vi "Indexer.vi"() -> ()   [LabVIEW 2020]
doc: "Use this template to build a producer/consumer design pattern with events to produce queue items. Use this design pattern instead of the User Interface Event Handler pattern for user interfaces when you want to execute code asynchronously in response to an event without slowing the user interface responsiveness."
uses:
  Model/AbstractModel/AbstractModel.lvclass
  Model/MarkovModel/MarkovModel.lvclass
  C:/Projects/DMC/DMC-Complete/Model/AbstractModel/AbstractModel.lvclass
  Indexer Action.ctl
  File Metadata.ctl
  Node.ctl
  Source to Sink Array.ctl
  File Data.ctl
panel:
  out "data":T5
  in  "Tab Control":enum32{"Main", "Debug"}(tab)
  out "# of files":i32 format="%d files"
  out "Markov Progress":u64(slide) scale=-1.0..127701.0
  out "Saving model to file":bool
  in  "Run Training":bool
  in  "Training Folders":path[](array[path])
  in  "Load Example Paths":bool
  out "Pulling training files":bool
  out "Converting to node-child maps":bool
  out "Training model":bool
  out "Node Progress":u64(slide) scale=-1.0..1339.0
  in  "stop":bool
  in  "Load from file":bool
  in  "Save to file":bool
  in  "Stage 3 - Train Model":bool
  in  "Stage 1 - Pull Example Files":bool
  in  "Stage 2 - Convert to Node-Child Maps":bool
  in  "Parallel Instances":i32=8
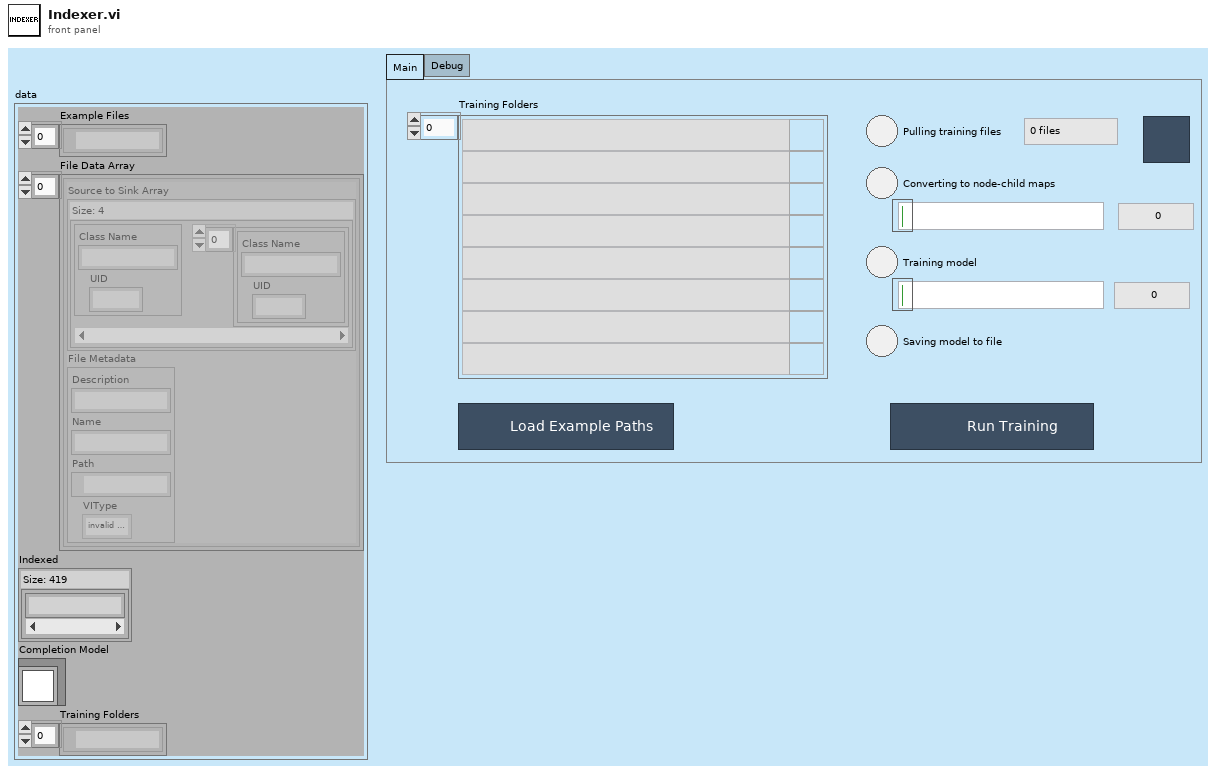
[diagram p1: front panel]
types:
  T1 = typedef "File Data.ctl" = cluster{"Source to Sink Array":T2, "File Metadata":T4}
  T2 = typedef "Source to Sink Array.ctl" = map{T3, T3[]}
  T3 = typedef "Node.ctl" = cluster{"Class Name":string, "UID":i32}
  T4 = typedef "File Metadata.ctl" = cluster{"Description":string, "Name":string, "Path":path, "VIType":enum32{"invalid VI type", "Standard VI", "Control VI", "Global VI", "Polymorphic VI", "Configuration VI", "SubSystem", "Facade VI", "Method VI", "Statechart Diagram VI"}}
  T5 = cluster{"Example Files":path[], "File Data Array":T1[], "Indexed":set{string}, "Completion Model":refnum<class "AbstractModel.lvclass">, "Training Folders":path[]}
  T6 = typedef "Indexer Action.ctl" = enum16{"Pull Training Files", "Convert to Node-Child Maps", "Train Model", "Save to file", "Load from file", "Load Example Paths"}
  T7 = enum8{"Enabled", "Disabled", "Disabled and Grayed Out"}
  T8 = cluster{"Example Files":path[], "File Data Array":T1[], "Indexed":set{string}, "MarkovModel out":refnum<class "MarkovModel.lvclass">, "Training Folders":path[]}
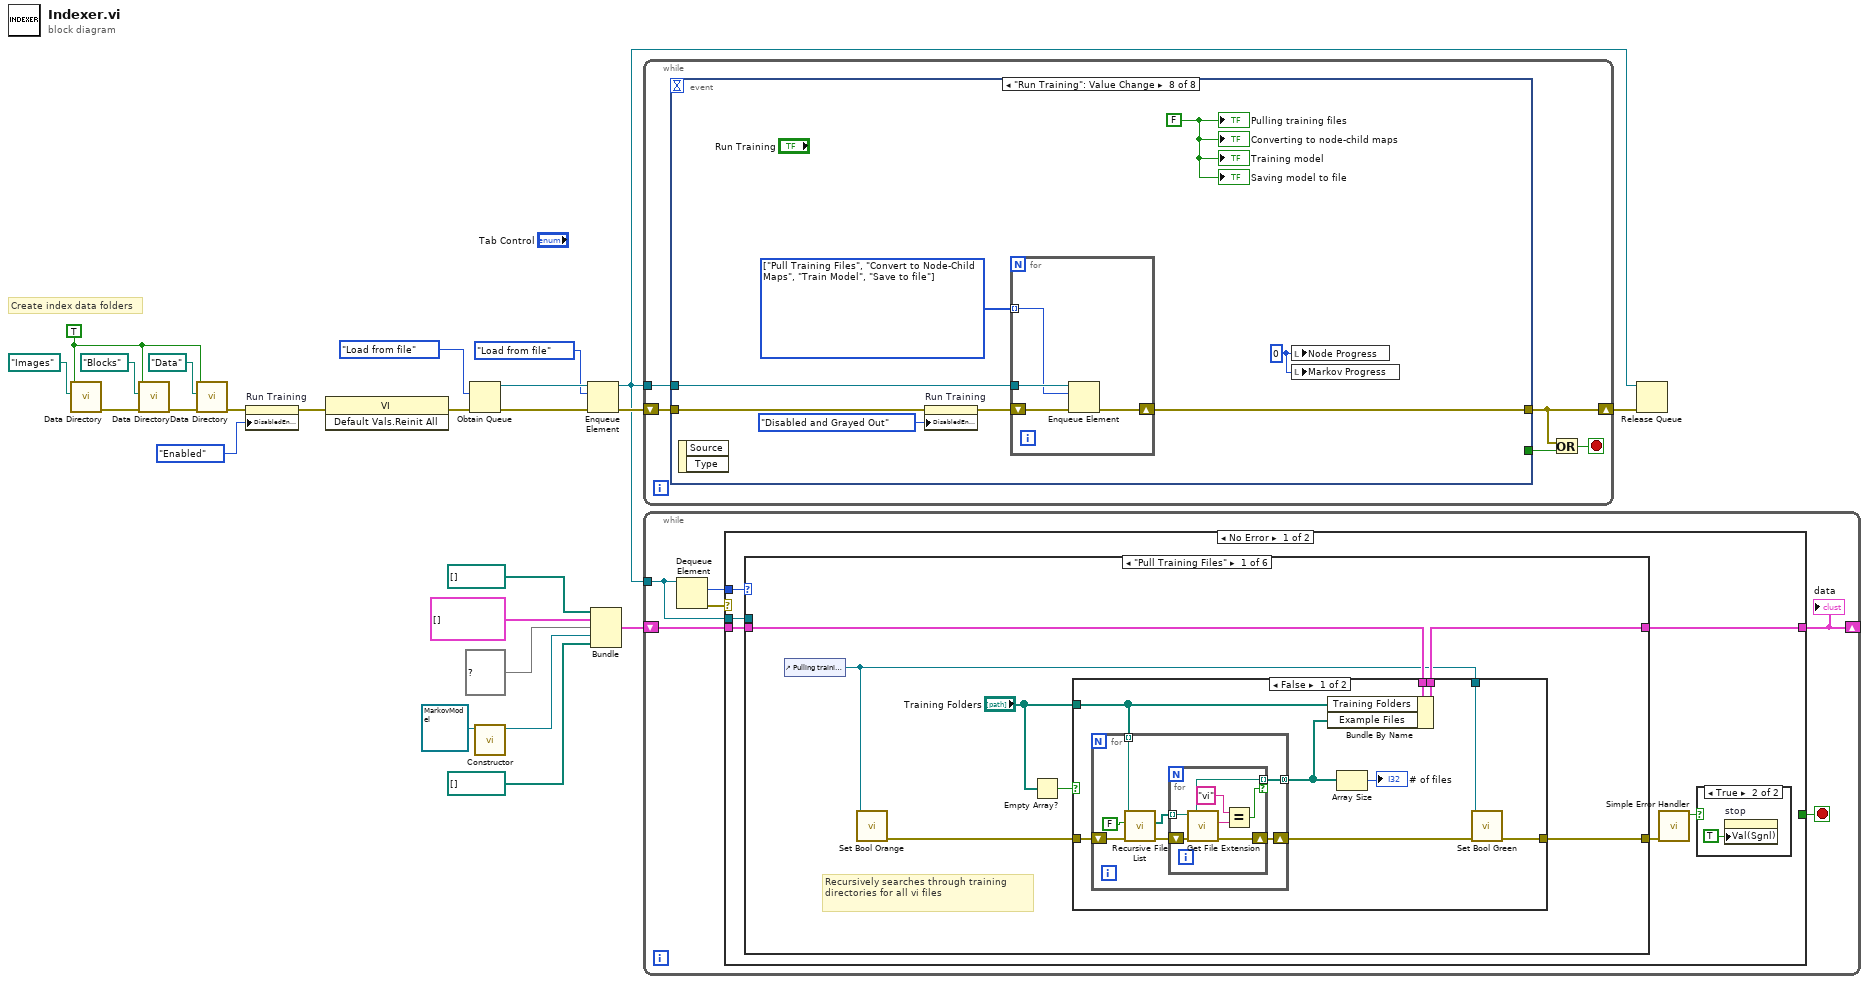
[diagram p0: block diagram]
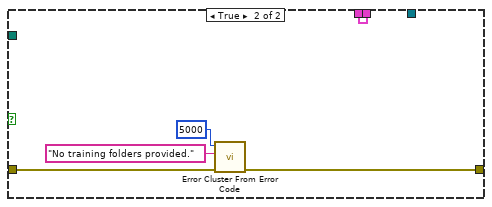
[diagram p2: hidden frame]
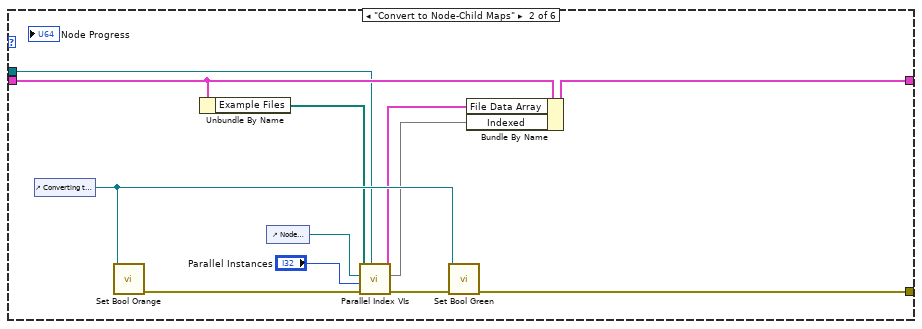
[diagram p3: hidden frame]
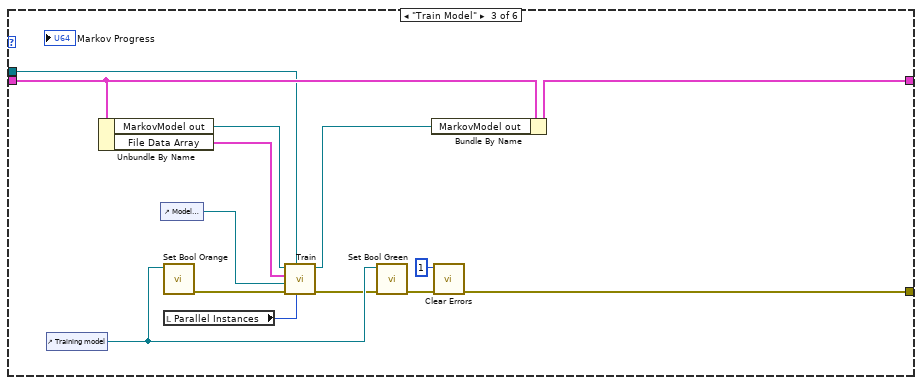
[diagram p4: hidden frame]
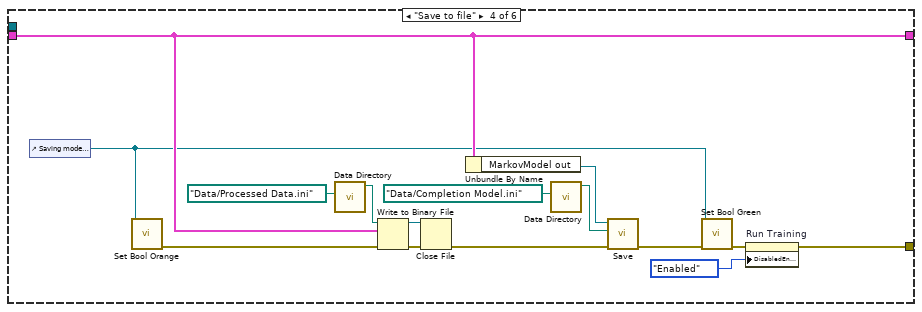
[diagram p5: hidden frame]
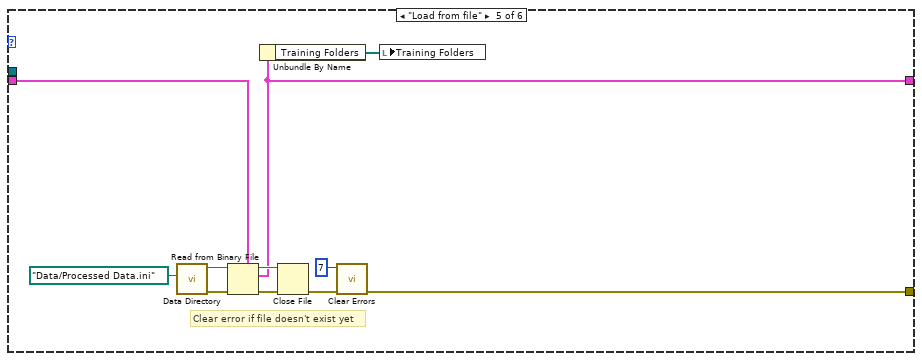
[diagram p6: hidden frame]
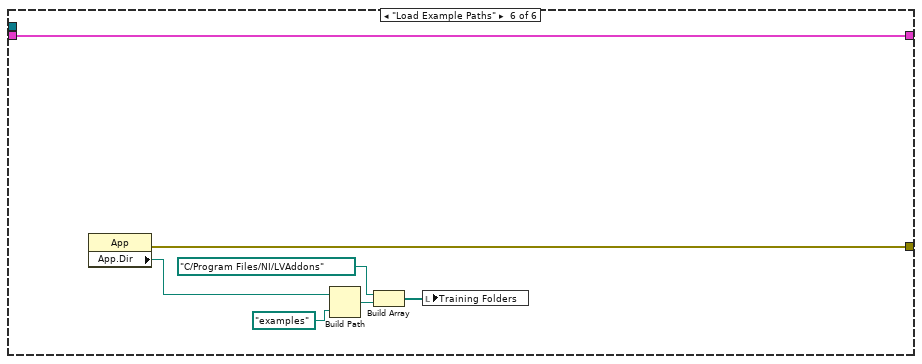
[diagram p7: hidden frame]
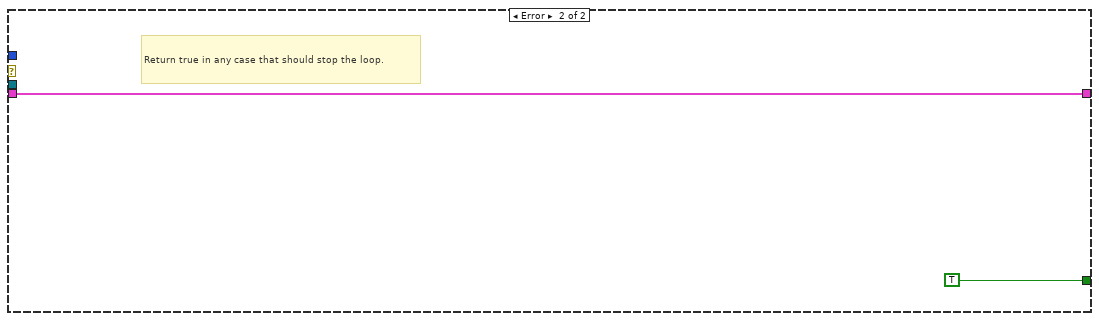
[diagram p9: hidden frame]
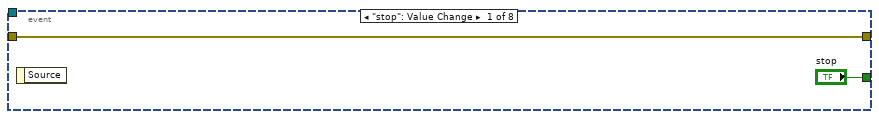
[diagram p10: hidden frame]
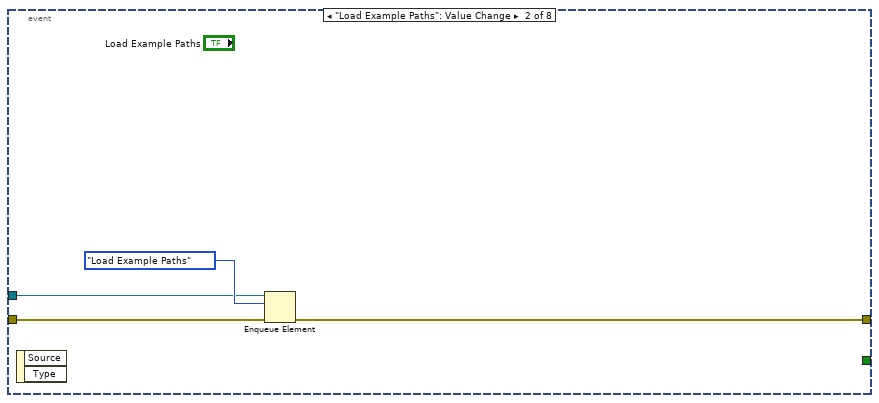
[diagram p11: hidden frame]
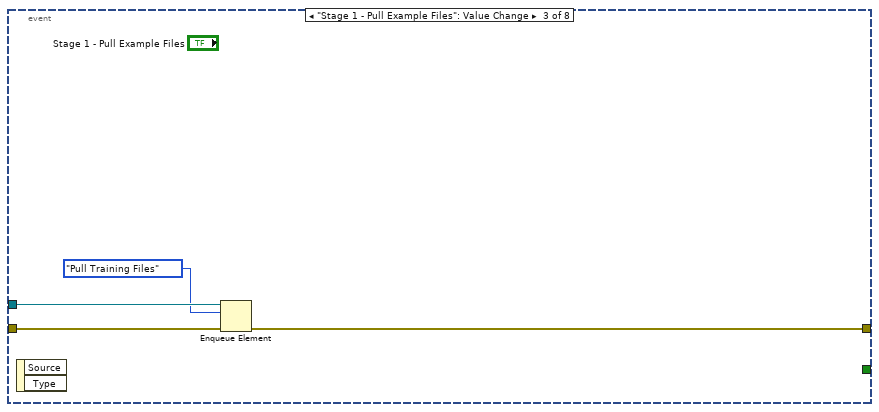
[diagram p12: hidden frame]
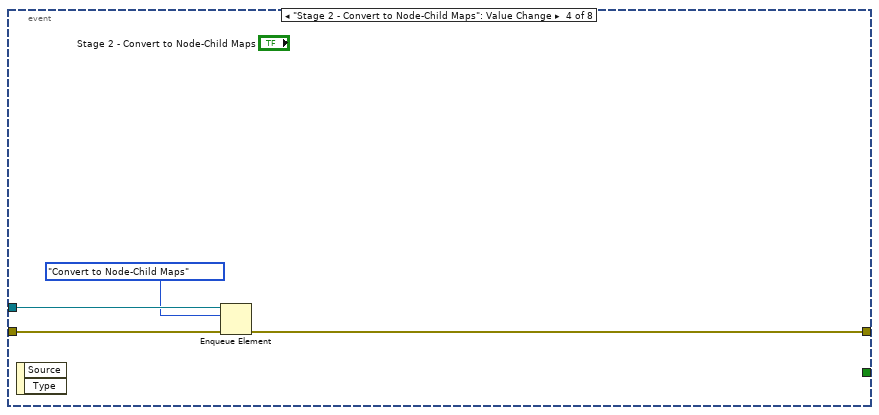
[diagram p13: hidden frame]
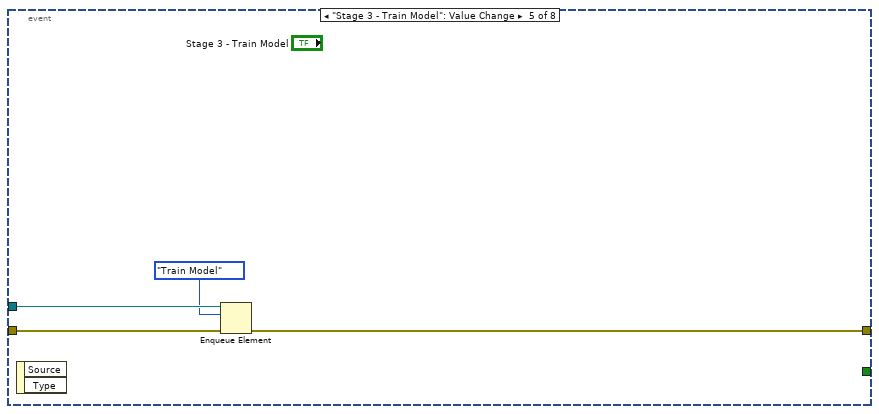
[diagram p14: hidden frame]
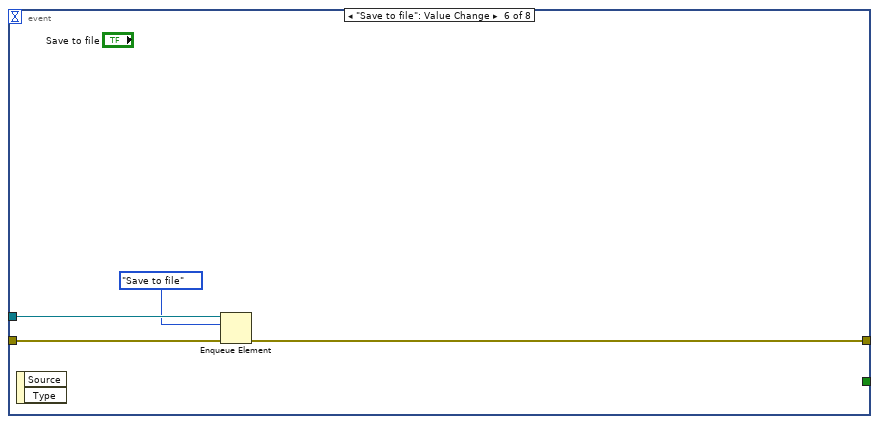
[diagram p15: hidden frame]
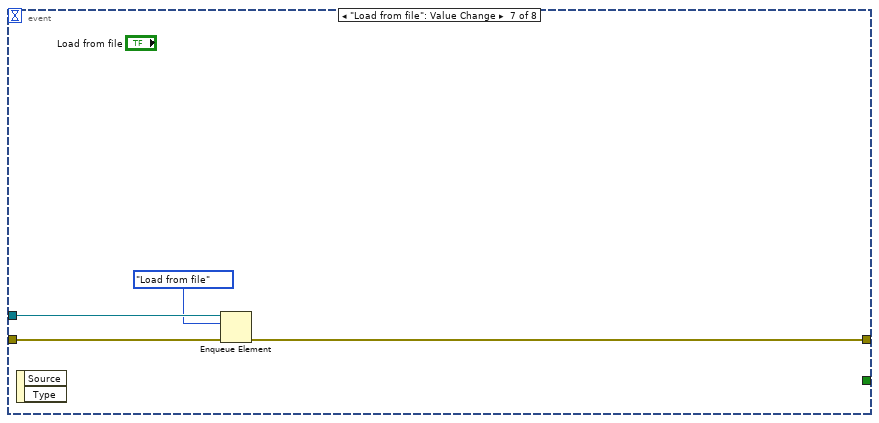
[diagram p16: hidden frame]
diagram:
  w5 = TRUE ("Create if doesn't exist? (F)")
  # "Create index data folders"
  n1 = call "Data Directory.vi"("Subdirectory"=path "Images" ("name or relative path"), "Create if doesn't exist? (F)"=w5) -> ("error out"=w6:errorcluster)  [unwired: 8 in, 1 out]
  n2 = call "Data Directory.vi"("error in (no error)"=w6, "Subdirectory"=path "Blocks" ("name or relative path"), "Create if doesn't exist? (F)"=w5) -> ("error out"=w7:errorcluster)  [unwired: 7 in, 1 out]
  n3 = call "Data Directory.vi"("error in (no error)"=w7, "Subdirectory"=path "Data" ("name or relative path"), "Create if doesn't exist? (F)"=w5) -> ("error out"=w4:errorcluster)  [unwired: 7 in, 1 out]
  n4 = property on="Run Training" class="Bool"(error in=w4, "DisabledEnum"=T7."Enabled") -> (error out=w12:errorcluster)  [unwired: 1 in, 1 out]
  n5 = invoke class="VI" method="Default Vals.Reinit All"(error in=w12) -> (error out=w14:errorcluster)  [unwired: 2 in, 2 out]
  n6 = Obtain Queue(element data type=Indexer_Action."Load from file" ("Indexer Action"), error in (no error)=w14) -> (queue out=w17:refnum<queue>, error out=w19:errorcluster)  [unwired: 3 in, 1 out]
  n7 = call-dynamic "Constructor.vi"("MarkovModel in"=refnum<class "MarkovModel.lvclass"> refnum ("MarkovModel.lvclass")) -> ("MarkovModel out"=w1:refnum<class "MarkovModel.lvclass">)  [unwired: 9 in, 1 out]
  n8 = Enqueue Element(queue=w17, element=Indexer_Action."Load from file", error in (no error)=w19) -> (queue out=w15:refnum<queue>, error out=w18:errorcluster)  [unwired: 1 in, 1 out]
  n9 = Bundle("Example Files"=path[] [], "File Data Array"=T1[] [], "Indexed"=set{string} {}, "MarkovModel out"=w1, "Training Folders"=path[] []) -> (w20:T8)  [unwired: 1 in]
  n10 = while {
    shift-right: [w25] -> w24
    shift-left: w18 -> [w28]
    tunnel: w15 -> [w29]
    stop <- w26 stop-if-true
    n11 = event shown="[7] \"Run Training\": Value Change" {
      selector: _ -> [_ _ _ _ _ _ _ _]
      dyn-events: _ -> [_ _ _ _ _ _ _ _]
      timeout: _ -> [_ _ _ _ _ _ _ _]
      tunnel: w29 -> [_ w32 w38 w42 w46 w50 w54 w63]
      tunnel: w28 -> [w30 w34 w39 w43 w47 w51 w55 w59]
      tunnel: [w30 w33 w37 w41 w45 w49 w53 w62] -> w25
      tunnel: ["stop" _ _ _ _ _ _ _] -> w27
      event "stop": Value Change {
        n12 = event-data() -> ()  [unwired: 1 in, 1 out]
      }
      event "Load Example Paths": Value Change {
        n13 = event-data() -> ()  [unwired: 1 in, 2 out]
        n14 = Enqueue Element(queue=w32, element=Indexer_Action."Load Example Paths" ("Indexer Action"), error in (no error)=w34) -> (error out=w33:errorcluster)  [unwired: 1 in, 2 out]
      }
      event "Stage 1 - Pull Example Files": Value Change {
        n15 = event-data() -> ()  [unwired: 1 in, 2 out]
        n16 = Enqueue Element(queue=w38, element=Indexer_Action."Pull Training Files" ("Indexer Action"), error in (no error)=w39) -> (error out=w37:errorcluster)  [unwired: 1 in, 2 out]
      }
      event "Stage 2 - Convert to Node-Child Maps": Value Change {
        n17 = event-data() -> ()  [unwired: 1 in, 2 out]
        n18 = Enqueue Element(queue=w42, element=Indexer_Action."Convert to Node-Child Maps" ("Indexer Action"), error in (no error)=w43) -> (error out=w41:errorcluster)  [unwired: 1 in, 2 out]
      }
      event "Stage 3 - Train Model": Value Change {
        n19 = event-data() -> ()  [unwired: 1 in, 2 out]
        n20 = Enqueue Element(queue=w46, element=Indexer_Action."Train Model" ("Indexer Action"), error in (no error)=w47) -> (error out=w45:errorcluster)  [unwired: 1 in, 2 out]
      }
      event "Save to file": Value Change {
        n21 = event-data() -> ()  [unwired: 1 in, 2 out]
        n22 = Enqueue Element(queue=w50, element=Indexer_Action."Save to file" ("Indexer Action"), error in (no error)=w51) -> (error out=w49:errorcluster)  [unwired: 1 in, 2 out]
      }
      event "Load from file": Value Change {
        n23 = event-data() -> ()  [unwired: 1 in, 2 out]
        n24 = Enqueue Element(queue=w54, element=Indexer_Action."Load from file" ("Indexer Action"), error in (no error)=w55) -> (error out=w53:errorcluster)  [unwired: 1 in, 2 out]
      }
      event "Run Training": Value Change {
        w56 = u64 0 ("Node Progress")
        w57 = FALSE ("Pulling training files")
        w61 = T6[] [enum."Pull Training Files", enum."Convert to Node-Child Maps", enum."Train Model", enum."Save to file"] items=["Pull Training Files", "Convert to Node-Child Maps", "Train Model", "Save to file", "Load from file", "Load Example Paths"] ("Array")
        n25 = event-data() -> ()  [unwired: 1 in, 2 out]
        n26 = property on="Run Training" class="Bool"(error in=w59, "DisabledEnum"=T7."Disabled and Grayed Out" ("Disabled")) -> (error out=w60:errorcluster)  [unwired: 1 in, 1 out]
        n27 = for {
          tunnel: w63 -> [w66]
          tunnel: w61 -> [w64] mode=indexing
          shift-right: [w65] -> w62
          shift-left: w60 -> [w67]
          n28 = Enqueue Element(queue=w66, element=w64, error in (no error)=w67) -> (error out=w65:errorcluster)  [unwired: 1 in, 2 out]
        }
        n29 = local write "Node Progress"(w56) -> ()
        n30 = local write "Markov Progress"(w56) -> ()
        "Converting to node-child maps" <- w57
        "Training model" <- w57
        "Pulling training files" <- w57
        "Saving model to file" <- w57
      }
    }
    n31 = Or(x=w25, y=w27) -> (x .or. y?=w26:bool)
  }
  n32 = while {
    tunnel: w15 -> [w69]
    shift-right: [w68] -> _
    shift-left: w20 -> [w70]
    stop <- w71 stop-if-true
    n33 = Dequeue Element(queue=w69) -> (element=w72:T6, error out=w73:errorcluster)  [unwired: 2 in, 2 out]
    n34 = case shown="No Error" w73 {
      tunnel: w72 -> [w79 _]
      tunnel: [_ TRUE] -> w71
      tunnel: w70 -> [w78 w174]
      tunnel: [w77 w174] -> w68
      tunnel: w69 -> [w76 _]
      frame No Error {
        n35 = case shown="\"Pull Training Files\"" w79 {
          tunnel: [w85 w125 w139 w152 w155 w167] -> w77
          tunnel: w78 -> [w86 w124 w137 w152 w163 w167]
          tunnel: w76 -> [_ w118 w131 _ _ _]
          tunnel: [w83 w122 w135 w147 w157 w168] -> w75
          frame "Pull Training Files" {
            # "Recursively searches through training directories for all vi files"
            n36 = control-ref of="Pulling training files"() -> (w82:refnum<vi>)
            n37 = call "Set Bool Orange.vi"("Indicator ref in"=w82) -> ("error out"=w84:errorcluster)  [unwired: 10 in]
            n38 = Empty Array?(array="Training Folders") -> (empty?=w80:bool)
            n39 = case shown="False" w80 {
              tunnel: w86 -> [w95 w113]
              tunnel: [w94 w113] -> w85
              tunnel: w84 -> [w93 w112]
              tunnel: [w91 w111] -> w83
              tunnel: w82 -> [w90 _]
              tunnel: "Training Folders" -> [w87 _]
              frame False {
                n40 = for {
                  tunnel: w87 -> [w102] mode=indexing
                  shift-right: [w97] -> w92
                  shift-left: w93 -> [w98]
                  tunnel: [w96] -> w89 mode=concatenating
                  n41 = call <vilib>:"Recursive File List.vi"("error in (no error)"=w98, "Treat LLBs as Folders?"=FALSE, "Folder Path"=w102) -> ("error out"=w99:errorcluster, "All Files in Dir"=w100:path[])  [unwired: 4 in, 3 out]
                  n42 = for {
                    tunnel: w100 -> [w105] mode=indexing
                    tunnel: [w105] -> w96 mode=indexing if=w104
                    shift-right: [w103] -> w97
                    shift-left: w99 -> [w108]
                    n43 = call <vilib>:"Get File Extension.vi"("error in (no error)"=w108, "file"=w105) -> ("error out"=w103:errorcluster, "lowercase file extension"=w106:string)  [unwired: 5 in, 3 out]
                    n44 = Equal?(x="vi", y=w106) -> (x = y?=w104:bool)
                  }
                }
                n45 = Bundle By Name(cluster=w95, "Training Folders"=w87, "Example Files"=w89) -> (w94:T8)
                n46 = Array Size(array=w89) -> (size(s)=→"# of files":i32)
                n47 = call "Set Bool Green.vi"("error in (no error)"=w92, "Indicator ref in"=w90) -> ("error out"=w91:errorcluster)  [unwired: 9 in]
              }
              frame True {
                n48 = call <vilib>:"Error Cluster From Error Code.vi"("error in (no error)"=w112, "error message (\"\")"="No training folders provided." ("error message (\"\")"), "error code (0)"=5000) -> ("error out"=w111:errorcluster)  [unwired: 6 in]
              }
            }
          }
          frame "Convert to Node-Child Maps" {
            n49 = control-ref of="Converting to node-child maps"() -> (w121:refnum<vi>)
            n50 = call "Set Bool Orange.vi"("Indicator ref in"=w121) -> ("error out"=w123:errorcluster)  [unwired: 10 in]
            n51 = Unbundle By Name(w124) -> ("Example Files"=w119:path[])
            n52 = control-ref of="Node Progress"() -> (w117:refnum<vi>)
            n53 = call "Parallel Index VIs.vi"("Queue in"=w118, "error in (no error)"=w123, "Parallel Instances (8)"="Parallel Instances", "Node Progress ref"=w117, "Example Files"=w119) -> ("error out"=w120:errorcluster, "Indexed"=w116:set{string}, "File Data Array"=w114:T1[])  [unwired: 4 in]
            n54 = call "Set Bool Green.vi"("error in (no error)"=w120, "Indicator ref in"=w121) -> ("error out"=w122:errorcluster)  [unwired: 9 in]
            n55 = Bundle By Name(cluster=w124, "File Data Array"=w114, "Indexed"=w116) -> (w125:T8)
          }
          frame "Train Model" {
            n56 = control-ref of="Training model"() -> (w138:refnum<vi>)
            n57 = Unbundle By Name(w137) -> ("MarkovModel out"=w130:refnum<class "MarkovModel.lvclass">, "File Data Array"=w129:T1[])
            n58 = control-ref of="Model Progress"() -> (w128:refnum<vi>)
            n59 = call "Set Bool Orange.vi"("Indicator ref in"=w138) -> ("error out"=w133:errorcluster)  [unwired: 10 in]
            n60 = local read "Parallel Instances"() -> (w127:i32)
            n61 = call-dynamic "Train.vi"("Parallel Instances (8)"=w127, "Queue in"=w131, "error in (no error)"=w133, "Progress ref in"=w128, "File Data Array"=w129, "MarkovModel in"=w130) -> ("error out"=w132:errorcluster, "MarkovModel out"=w126:refnum<class "MarkovModel.lvclass">)  [unwired: 4 in]
            n62 = call "Set Bool Green.vi"("error in (no error)"=w132, "Indicator ref in"=w138) -> ("error out"=w136:errorcluster)  [unwired: 9 in]
            n63 = Bundle By Name(cluster=w137, "MarkovModel out"=w126) -> (w139:T8)
            n64 = call <vilib>:"Clear Errors.vi"("error in (no error)"=w136, "specific error code to clear (0: all)"=1) -> ("error out"=w135:errorcluster)  [unwired: 4 in, 1 out]
          }
          frame "Save to file" {
            n65 = control-ref of="Saving model to file"() -> (w150:refnum<vi>)
            n66 = call "Set Bool Orange.vi"("Indicator ref in"=w150) -> ("error out"=w151:errorcluster)  [unwired: 10 in]
            n67 = call "Data Directory.vi"("Subdirectory"=path "Data/Processed Data.ini" ("name or relative path")) -> ("Data directory"=w145:path)  [unwired: 9 in, 1 out]
            n68 = Write to Binary File(file (use dialog)=w145, data=w152, error in=w151) -> (refnum out=w153:refnum<file>, error out=w154:errorcluster)  [unwired: 3 in, 1 out]
            n69 = Close File(refnum=w153, error in=w154) -> (error out=w144:errorcluster)  [unwired: 1 out]
            n70 = Unbundle By Name(w152) -> ("MarkovModel out"=w142:refnum<class "MarkovModel.lvclass">)
            n71 = call "Data Directory.vi"("Subdirectory"=path "Data/Completion Model.ini" ("name or relative path")) -> ("Data directory"=w140:path)  [unwired: 9 in, 1 out]
            n72 = call-dynamic "Save.vi"("error in (no error)"=w144, "Model Path"=w140, "MarkovModel in"=w142) -> ("error out"=w143:errorcluster)  [unwired: 7 in, 1 out]
            n73 = call "Set Bool Green.vi"("error in (no error)"=w143, "Indicator ref in"=w150) -> ("error out"=w148:errorcluster)  [unwired: 9 in]
            n74 = property on="Run Training" class="Bool"(error in=w148, "DisabledEnum"=T7."Enabled" ("Disabled")) -> (error out=w147:errorcluster)  [unwired: 1 in, 1 out]
          }
          frame "Load from file" {
            # "Clear error if file doesn't exist yet"
            n75 = call "Data Directory.vi"("Subdirectory"=path "Data/Processed Data.ini" ("name or relative path")) -> ("error out"=w156:errorcluster, "Data directory"=w158:path)  [unwired: 9 in]
            n76 = Read from Binary File(5:w163, 8:w156, 11:w158) -> (0:w165:errorcluster, 2:w155:T8, 3:w164:refnum<file>)  [unwired: 3 in, 1 out]
            n77 = Unbundle By Name(w155) -> ("Training Folders"=w162:path[])
            n78 = Close File(refnum=w164, error in=w165) -> (error out=w161:errorcluster)  [unwired: 1 out]
            n79 = call <vilib>:"Clear Errors.vi"("error in (no error)"=w161, "specific error code to clear (0: all)"=7) -> ("error out"=w157:errorcluster)  [unwired: 4 in, 1 out]
            n80 = local write "Training Folders"(w162) -> ()
          }
          frame "Load Example Paths" {
            n81 = property class="App"() -> (error out=w168:errorcluster, "App.Dir"=w169:path)  [unwired: 2 in, 1 out]
            n82 = Build Path(base path=w169, name or relative path=path "examples" ("Path")) -> (appended path=w170:path)
            n83 = Build Array(path "C:/Program Files/NI/LVAddons" ("Path"), w170) -> (w166:path[])
            n84 = local write "Training Folders"(w166) -> ()
          }
        }
        n85 = call <vilib>:"Simple Error Handler.vi"("error in (no error)"=w75) -> ("error?"=w74:bool)  [unwired: 4 in, 4 out]
        n86 = case shown="True" w74 {
          frame False {
          }
          frame True {
            n87 = property on="stop" class="Bool (strict)"("Val(Sgnl)"=TRUE ("Value (Signaling)")) -> ()  [unwired: 2 in, 2 out]
          }
        }
      }
      frame Error {
        # "Return true in any case that should stop the loop."
      }
    }
    "data" <- w68
  }
  n88 = Release Queue(queue=w15, error in (no error)=w24) -> ()  [unwired: 1 in, 3 out]
